vi "HFRR ADV v037 new software.vi"() -> ()   [LabVIEW 2025] (continued)
              n2898 = local write "Numeric 16"(w3970) -> ()
              n2899 = String Length(string=w3972) -> (length=w3975:i32)
              n2900 = Greater?(x=w3975, y=1) -> (0:w3971:bool)
            }
            n2901 = local write "String 29"(w3952) -> ()
            n2902 = Search and Replace String(input string=w3952, search string=".duf", replace string=".dgf" ("replace string (\"\")")) -> (result string=→"String Indicator 4":string)  [unwired: 5 in, 3 out]
            n2903 = Match Pattern(string=w3967, regular expression=".dwm") -> (before substring=w3951:string)  [unwired: 1 in, 3 out]
            "String Indicator" <- w3951
            n2904 = Match Pattern(string=w3952, regular expression=".dwm" ("substring (\"\")")) -> (before substring=w3953:string)  [unwired: 1 in, 3 out]
            "String Indicator 3" <- w3953
            n2905 = local write "TITTLE 2"(w3951) -> ()
            n2906 = String To Path(string=w3953) -> (path=w3960:path)
            "path" <- w3960
            n2907 = call <vilib>:"Read Characters From File.vi"("file path (dialog if empty)"=w3960, "start of read offset (chars.:0)"=60 ("start of read offset (chars.: 0)")) -> ("character string"=→"String Indicator 2":string)  [unwired: 4 in, 3 out]
          }
        }
        n2908 = call <vilib>:"Query Available Printers.vi"() -> ("system configured printers"=w3652:string[])  [unwired: 9 in, 2 out]
        "System Configured Printers 2" <- w3652
        n2909 = local read "OK Button 16"() -> (w3649:bool)
        n2910 = case shown="True" "OK Button 16" {
          frame False {
          }
          frame True {
            n2911 = stacked-sequence {
              frame #0 {
                n2912 = local read "Numeric 16"() -> (w3977:i32)
                n2913 = local write "Numeric 10"(w3977) -> ()
              }
              frame #1 {
                n2914 = local read "String 29"() -> (w3980:string)
                n2915 = String To Path(string=w3980) -> (path=w3979:path)
                n2916 = Open/Create/Replace File "Open File"(file path (use dialog)=w3979) -> (refnum out=w3981:refnum<file>)  [unwired: 5 in, 2 out]
                n2917 = for {
                  N: 16 -> [_]
                  tunnel: w3981 -> [w3988]
                  i -> [w3984]
                  (unwired) TRUE ("line mode (F)")
                  n2918 = Read from Text File "Read File"(file (use dialog)=w3988) -> (text=w3982:string)  [unwired: 3 in, 3 out]
                  n2919 = Match Pattern(string=w3982, regular expression="(") -> (after substring=w3987:string)  [unwired: 1 in, 3 out]
                  n2920 = Match Pattern(string=w3987, regular expression=")") -> (before substring=w3983:string)  [unwired: 1 in, 3 out]
                  n2921 = case shown="1" w3984 {
                    tunnel: w3983 -> [w3989 w3990 _ _ w3991 w3992 w3993 w3995 w3997 w3999 w4001 w4003 w4005 w4007 _]
                    tunnel: w3982 -> [_ _ _ _ _ _ _ _ _ _ _ _ _ _ _]
                    frame 0 {
                      "TITTLE" <- w3989
                    }
                    frame 1 {
                      "Sample ID" <- w3990
                    }
                    frame 2 {
                    }
                    frame 3 {
                    }
                    frame 4 {
                      "Test Date" <- w3991
                    }
                    frame 5 {
                      "Tested by" <- w3992
                    }
                    frame 6 {
                      n2922 = Fract/Exp String To Number(string=w3993) -> (number=→"Humidity before test 2":dbl)  [unwired: 3 in, 1 out]
                    }
                    frame 7 {
                      n2923 = Fract/Exp String To Number(string=w3995) -> (number=→"Temperature before test 2":dbl)  [unwired: 3 in, 1 out]
                    }
                    frame 8 {
                      n2924 = Fract/Exp String To Number(string=w3997) -> (number=→"Humidity after test 2":dbl)  [unwired: 3 in, 1 out]
                    }
                    frame 9 {
                      n2925 = Fract/Exp String To Number(string=w3999) -> (number=→"Temperature after test 2":dbl)  [unwired: 3 in, 1 out]
                    }
                    frame 10 {
                      n2926 = Fract/Exp String To Number(string=w4001) -> (number=→"MWSD 2":dbl)  [unwired: 3 in, 1 out]
                    }
                    frame 11 {
                      n2927 = Fract/Exp String To Number(string=w4003) -> (number=→"AVP 2":dbl)  [unwired: 3 in, 1 out]
                    }
                    frame 12 {
                      n2928 = Fract/Exp String To Number(string=w4005) -> (number=→"HCF 2":dbl)  [unwired: 3 in, 1 out]
                    }
                    frame 13 {
                      n2929 = Fract/Exp String To Number(string=w4007) -> (number=→"WS1.4 2":dbl)  [unwired: 3 in, 1 out]
                    }
                    frame 14, Default {
                    }
                  }
                }
              }
              frame #2 {
              }
            }
            n2930 = local write "OK Button 16"(FALSE ("OK Button 13")) -> ()
          }
        }
        n2931 = Index Array(array=w3652, index="Select Printer 3") -> (element=w3654:string)
        "Selected Printer" <- w3654
        n2932 = case shown="True" w3649 {
          frame False {
          }
          frame True {
            n2933 = flat-sequence {
              frame #0 {
              }
              frame #1 {
                n2934 = Wait (ms)(milliseconds to wait=u32 100) -> ()  [unwired: 1 out]
              }
              frame #2 {
                n2935 = local write "OK Button 16"(FALSE ("Print 3")) -> ()
              }
            }
          }
        }
        n2936 = case shown="True" "Print" {
          tunnel: w3654 -> [_ w3946]
          frame False {
          }
          frame True {
            (unwired) i16 6 ("width (-)")
            (unwired) "TESTED BY : "
            (unwired) "TESTED DATE :"
            (unwired) "SAMPLE ID : "
            (unwired) "SAMPLE DESIGN : "
            w3904 = "\r"
            w3921 = "\r"
            # "add image"
            n2937 = local read "Sample ID"() -> (w3894:string)
            n2938 = local read "Tested by"() -> (w3897:string)
            n2939 = local read "String 34"() -> (w3884:string)
            n2940 = local read "String 45"() -> (w3864:string)
            n2941 = local read "String 35"() -> (w3879:string)
            n2942 = local read "String 37"() -> (w3877:string)
            n2943 = local read "String 32"() -> (w3899:string)
            n2944 = local read "String 36"() -> (w3874:string)
            n2945 = local read "String 31"() -> (w3898:string)
            n2946 = local read "Test Date"() -> (w3895:string)
            n2947 = local read "String 33"() -> (w3900:string)
            n2948 = local read "String 38"() -> (w3870:string)
            n2949 = local read "String 39"() -> (w3867:string)
            n2950 = local write "Print"(FALSE ("Print FF")) -> ()
            n2951 = local read "S 39"() -> (w3882:string)
            n2952 = local read "S 38"() -> (w3889:string)
            n2953 = local read "Temperature before test 2"() -> (w3920:dbl)
            n2954 = local read "Temperature after test 2"() -> (w3910:dbl)
            n2955 = local read "Humidity before test 2"() -> (w3935:dbl)
            n2956 = local read "Humidity after test 2"() -> (w3919:dbl)
            n2957 = local read "MWSD 2"() -> (w3924:dbl)
            n2958 = local read "WS1.4 2"() -> (w3902:dbl)
            n2959 = Concatenate Strings("2)" ("string"), w3884) -> (w3885:string)
            n2960 = Concatenate Strings("3)" ("string"), w3882) -> (w3883:string)
            n2961 = Concatenate Strings("1)" ("string"), w3889) -> (w3888:string)
            n2962 = Concatenate Strings("4)" ("string"), w3879) -> (w3880:string)
            n2963 = Concatenate Strings("5)" ("string"), w3877) -> (w3876:string)
            n2964 = Concatenate Strings("6)" ("string"), w3874) -> (w3873:string)
            n2965 = Concatenate Strings("7)" ("string"), w3870) -> (w3871:string)
            n2966 = Concatenate Strings("8)" ("string"), w3867) -> (w3868:string)
            n2967 = local read "HCF 2"() -> (w3906:dbl)
            n2968 = local read "AVP 2"() -> (w3923:dbl)
            n2969 = local read "s.NO"() -> (w3865:string)
            n2970 = call <vilib>:"New Report.vi"("report type"=enum16{"Standard Report", "HTML"}."Standard Report") -> ("report out"=w3944:refnum<class "NI_report.lvclass">, "error out"=w3943:errorcluster)  [unwired: 13 in]
            n2971 = local read "TITTLE"() -> (w3896:string)
            n2972 = Concatenate Strings(w3921, w3864, w3865, w3921, w3899, w3894, w3921, w3898, w3895, w3921, w3900, w3897, w3921) -> (w3914:string)
            "test by" <- w3914
            n2973 = Number To Fractional String(number=w3920, width (-)=i16 6, precision (6)=i16 2) -> (F-format string=w3909:string)  [unwired: 1 in]
            n2974 = Number To Fractional String(number=w3919, width (-)=i16 6, precision (6)=i16 2) -> (F-format string=w3922:string)  [unwired: 1 in]
            n2975 = Number To Fractional String(number=w3935, width (-)=i16 6, precision (6)=i16 2) -> (F-format string=w3940:string)  [unwired: 1 in]
            n2976 = Number To Fractional String(number=w3924, width (-)=i16 6, precision (6)=i16 2) -> (F-format string=w3926:string)  [unwired: 1 in]
            n2977 = Number To Fractional String(number=w3910, width (-)=i16 6, precision (6)=i16 2) -> (F-format string=w3911:string)  [unwired: 1 in]
            n2978 = Number To Fractional String(number=w3923, width (-)=i16 6, precision (6)=i16 2) -> (F-format string=w3925:string)  [unwired: 1 in]
            n2979 = Number To Fractional String(number=w3906, width (-)=i16 6, precision (6)=i16 2) -> (F-format string=w3905:string)  [unwired: 1 in]
            n2980 = Number To Fractional String(number=w3902, precision (6)=i16 2) -> (F-format string=w3901:string)  [unwired: 2 in]
            n2981 = call-dynamic "Set Report Header Text.vi"("report in"=w3944, "center header text"=w3896, "error in (no error)"=w3943) -> ("report out"=w3915:refnum<class "NI_report.lvclass">, "error out"=w3916:errorcluster)  [unwired: 11 in]
            n2982 = Concatenate Strings(w3904, w3888, w3940, w3904, w3885, w3909, w3904, w3883, w3922, w3904, w3880, w3911, w3904, w3876, w3926, w3904, w3873, w3925, w3904, w3871, w3905, w3904, w3868, w3901) -> (w3892:string)
            "export 2" <- w3892
            n2983 = call-poly <vilib>:"Append Report Text.vi"("report in"=w3915, "text"=w3914, "error in (no error)"=w3916) -> ("report out"=w3918:refnum<class "NI_report.lvclass">, "error out"=w3917:errorcluster)  [unwired: 9 in, 2 out]
            n2984 = local read "test by"() -> (w3891:string)
            n2985 = local read "TITTLE"() -> (w3893:string)
            n2986 = call-poly <vilib>:"Append Report Text.vi"("report in"=w3918, "error in (no error)"=w3917) -> ("report out"=w3939:refnum<class "NI_report.lvclass">, "error out"=w3937:errorcluster)  [unwired: 10 in, 2 out]
            n2987 = Concatenate Strings(w3893, w3892, w3891) -> (→"output":string)
            n2988 = call-poly <vilib>:"Append Report Text.vi"("report in"=w3939, "text"=w3892, "error in (no error)"=w3937) -> ("report out"=w3938:refnum<class "NI_report.lvclass">, "error out"=w3936:errorcluster)  [unwired: 9 in, 2 out]
            n2989 = call-dynamic "Print Report.vi"("report in"=w3938, "printer name (default)"=w3946, "error in (no error)"=w3936) -> ("report out"=w3948:refnum<class "NI_report.lvclass">, "error out"=w3949:errorcluster)  [unwired: 11 in]
            n2990 = call-dynamic "Dispose Report.vi"("report in"=w3948, "error in (no error)"=w3949) -> ()  [unwired: 13 in, 1 out]
          }
        }
        n2991 = case shown="True" "Print 2" {
          frame False {
          }
          frame True {
            n2992 = flat-sequence {
              frame #0 {
                n2993 = local read "s.NO"() -> (→"s.NO 2":string)
                n2994 = Wait (ms)(milliseconds to wait=u32 20) -> ()  [unwired: 1 out]
                n2995 = local read "Sample ID  3"() -> (→"Sample ID  6":string)
                n2996 = local read "Sample ID  4"() -> (→"Sample ID  7":string)
                n2997 = local read "Sample ID"() -> (→"Sample ID  2":string)
                n2998 = local read "Tested by"() -> (→"Tested by 2":string)
                n2999 = local read "Test Date"() -> (→"Test Date 2":string)
                n3000 = local read "Humidity after test 3"() -> (→"Humidity after test 4":dbl)
                n3001 = local read "Ref A Test Date :"() -> (→"TITTLE 4":string)
                n3002 = local read "Temperature before test 3"() -> (w3771:dbl)
                n3003 = local read "Temperature before test 3"() -> (→"Temperature after test 5":dbl)
                n3004 = local read "Temperature after test 3"() -> (→"Temperature after test 4":dbl)
                n3005 = local read "Humidity before test 3"() -> (→"Humidity before test 4":dbl)
                n3006 = local write "Temperature before test 3"(w3771) -> ()
                n3007 = local read "image data"() -> (w3762:T16)
                n3008 = String To Path(string="C:\\LAB-IQ\\im\\Temp_resized.jpg") -> (path=w3763:path)
                "path 2" <- w3763
                n3009 = call <vilib>:"Write JPEG File.vi"("image data"=w3762, "path to JPEG file"=w3763) -> ()  [unwired: 8 in, 2 out]
                "Ref A Test Date :" <- "Ref A Test Date :"
                "Ref B Test Date :" <- "Ref B Test Date :"
                "Ref B Scar Value :" <- "Ref B Scar Value :"
                "Ref A Scar Value :" <- "Ref A Scar Value :"
              }
              frame #1 {
                (unwired) HTML_Report_Image_Alignment."MIDDLE" ("alignment (default)")
                w3799 = u16 0 items=["portrait", "landscape"] ("orientation (portrait)")
                (unwired) HTML_Report_Image_Alignment."ABSMIDDLE" ("alignment (default)")
                (unwired) "TESTED BY : "
                (unwired) "TESTED DATE :"
                (unwired) "SAMPLE ID : "
                (unwired) "SAMPLE DESIGN : "
                w3832 = "\r"
                # "add image"
                n3010 = Wait (ms)(milliseconds to wait=u32 20) -> ()  [unwired: 1 out]
                n3011 = local read "Sample ID  2"() -> (w3825:string)
                n3012 = local read "Wear Scar X"() -> (w3797:dbl)
                "Length ( microns ) 2" <- w3797
                n3013 = local read "Wear Scar Y"() -> (w3796:dbl)
                "Wear Scar Y ( microns ) :" <- w3796
                n3014 = local read "Test Date 2"() -> (w3826:string)
                n3015 = local read "Tested by 2"() -> (w3827:string)
                n3016 = local read "String 46"() -> (w3823:string)
                n3017 = local read "String 48"() -> (w3829:string)
                n3018 = local read "String 47"() -> (w3828:string)
                n3019 = local read "String 49"() -> (w3830:string)
                n3020 = local read "String 10"() -> (w3783:string)
                n3021 = local read "s.NO 2"() -> (w3824:string)
                n3022 = Add(x=w3797, y=w3796) -> (x+y=w3795:dbl)
                n3023 = call <vilib>:"New Report.vi"("report type"=enum16{"Standard Report", "HTML"}."HTML") -> ("report out"=w3803:refnum<class "NI_report.lvclass">, "error out"=w3801:errorcluster)  [unwired: 13 in]
                n3024 = Concatenate Strings(w3832, w3823, w3824, w3832, w3829, w3825, w3832, w3828, w3826, w3832, w3830, w3827, w3832) -> (→"test by 2":string)
                n3025 = Concatenate Strings("C:\\LAB-IQ\\Data\\" ("string"), w3783, ".jpg" ("string")) -> ()  [unwired: 1 out]
                n3026 = Divide(x=w3795, y=2.0) -> (x/y=→"Mean Wear ( microns) :":dbl)
                n3027 = call-dynamic "Set Report Orientation.vi"("report in"=w3803, "orientation (portrait)"=w3799, "error in (no error)"=w3801) -> ("report out"=w3802:refnum<class "NI_report.lvclass">, "error out"=w3800:errorcluster)  [unwired: 11 in]
                n3028 = for {
                  N: 5 -> [_]
                  tunnel: w3802 -> [w3853]
                  tunnel: [w3852] -> w3781
                  tunnel: w3800 -> [w3851]
                  tunnel: [w3850] -> w3780
                  n3029 = call-dynamic "Set Report Tab Width.vi"("report in"=w3853, "error in (no error)"=w3851) -> ("report out"=w3852:refnum<class "NI_report.lvclass">, "error out"=w3850:errorcluster)  [unwired: 12 in]
                }
                n3030 = local read "TITTLE"() -> (w3798:string)
                n3031 = call-dynamic "Set Report Header Text.vi"("report in"=w3781, "center header text"=w3798, "error in (no error)"=w3780) -> ("report out"=w3819:refnum<class "NI_report.lvclass">, "error out"=w3818:errorcluster)  [unwired: 11 in]
                n3032 = for {
                  N: 1 -> [_]
                  tunnel: [w3857] -> w3805
                  tunnel: [w3856] -> w3804
                  tunnel: w3819 -> [w3855]
                  tunnel: w3818 -> [w3854]
                  n3033 = call-dynamic "New Report Line.vi"("report in"=w3855, "error in (no error)"=w3854) -> ("report out"=w3857:refnum<class "NI_report.lvclass">, "error out"=w3856:errorcluster)  [unwired: 12 in]
                }
                n3034 = for {
                  N: 2 -> [_]
                  tunnel: [w3849] -> w3811
                  tunnel: [w3848] -> w3810
                  tunnel: w3805 -> [w3847]
                  tunnel: w3804 -> [w3846]
                  n3035 = call-dynamic "New Report Line.vi"("report in"=w3847, "error in (no error)"=w3846) -> ("report out"=w3849:refnum<class "NI_report.lvclass">, "error out"=w3848:errorcluster)  [unwired: 12 in]
                }
                n3036 = for {
                  N: 25 -> [_]
                  tunnel: w3811 -> [w3845]
                  tunnel: w3810 -> [w3843]
                  tunnel: [w3844] -> w3814
                  tunnel: [w3842] -> w3813
                  n3037 = call-dynamic "Set Report Tab Width.vi"("report in"=w3845, "error in (no error)"=w3843) -> ("report out"=w3844:refnum<class "NI_report.lvclass">, "error out"=w3842:errorcluster)  [unwired: 12 in]
                }
                n3038 = control-ref of="Tab Control 9"() -> (w3809:refnum<vi>)
                n3039 = call-dynamic "Append Control Image to Report.vi"("report in"=w3814, "alignment (default)"=HTML_Report_Image_Alignment."ABSMIDDLE", "ctrl reference"=w3809, "error in (no error)"=w3813) -> ("report out"=w3808:refnum<class "NI_report.lvclass">, "error out"=w3807:errorcluster)  [unwired: 8 in, 2 out]
                n3040 = for {
                  N: 3 -> [_]
                  tunnel: [w3841] -> w3792
                  tunnel: [w3840] -> w3791
                  tunnel: w3808 -> [w3839]
                  tunnel: w3807 -> [w3838]
                  n3041 = call-dynamic "New Report Line.vi"("report in"=w3839, "error in (no error)"=w3838) -> ("report out"=w3841:refnum<class "NI_report.lvclass">, "error out"=w3840:errorcluster)  [unwired: 12 in]
                }
                n3042 = for {
                  N: 100 -> [_]
                  tunnel: w3792 -> [w3837]
                  tunnel: w3791 -> [w3835]
                  tunnel: [w3836] -> w3788
                  tunnel: [w3834] -> w3786
                  n3043 = call-dynamic "Set Report Tab Width.vi"("report in"=w3837, "error in (no error)"=w3835) -> ("report out"=w3836:refnum<class "NI_report.lvclass">, "error out"=w3834:errorcluster)  [unwired: 12 in]
                }
                n3044 = String To Path(string="C:\\LAB-IQ\\im\\Temp_resized.jpg") -> (path=w3778:path)
                n3045 = call-poly <vilib>:"Append Image to Report.vi"("report in"=w3788, "path or URL of image"=w3778, "error in (no error)"=w3786) -> ("report out"=w3787:refnum<class "NI_report.lvclass">, "error out"=w3785:errorcluster)  [unwired: 9 in, 2 out]
                n3046 = call-poly <vilib>:"Open HTML Report in Browser.vi"("report in"=w3787, "error in (no error)"=w3785) -> ("report out"=w3822:refnum<class "NI_report.lvclass">, "error out"=w3821:errorcluster)  [unwired: 11 in, 1 out]
                n3047 = call-dynamic "Dispose Report.vi"("report in"=w3822, "error in (no error)"=w3821) -> ()  [unwired: 13 in, 1 out]
              }
              frame #2 {
              }
              frame #3 {
                n3048 = disable-structure shown="Disabled" {
                  frame Disabled {
                    n3049 = local read "String 10"() -> (w3862:string)
                    n3050 = Concatenate Strings("C:\\LAB-IQ-NXT\\Data\\" ("string"), w3862, ".jpg" ("string")) -> (w3860:string)
                    n3051 = String To Path(string=w3860) -> (path=w3859:path)
                    n3052 = Delete(path (use dialog)=w3859) -> ()  [unwired: 4 in, 3 out]
                  }
                  frame Enabled {
                  }
                }
                n3053 = local write "Print 2"(FALSE ("Print")) -> ()
              }
            }
          }
        }
      }
    }
    n3054 = Wait (ms)(milliseconds to wait=u32 50) -> ()  [unwired: 1 out]
    n3055 = Wait (ms)(milliseconds to wait=u32 50) -> ()  [unwired: 1 out]
    n3056 = local read "Quit"() -> (w2196:bool)
  }
  n3057 = VISA Close(VISA resource name=w41, error in (no error)=w40) -> ()  [unwired: 1 out]
  n3058 = while {
    stop <- w4013 stop-if-true
    n3059 = local read "Auto Start Test"() -> (w4011:bool)
    n3060 = local read "RUN"() -> (w4010:bool)
    n3061 = Wait (ms)(milliseconds to wait=u32 1000) -> ()  [unwired: 1 out]
    n3062 = Or(x=w4010, y=w4011) -> (x .or. y?=w4009:bool)
    n3063 = case shown="True" w4009 {
      frame False {
      }
      frame True {
        n3064 = local read "LVDT STROKE Actual"() -> (w4014:dbl)
        n3065 = In Range and Coerce(upper limit=1.2, x=w4014, lower limit=0.6) -> (In Range?=w4017:bool)  [unwired: 1 out]
        n3066 = call-poly <vilib>:"Random Number (Range).vi"("lower bound (0)"=0.998 ("upper bound (100)"), "upper bound (100)"=1.003) -> ("number"=w4015:dbl)  [unwired: 9 in]
        n3067 = case shown="True" w4017 {
          tunnel: [w4022 w4023] -> w4016
          tunnel: w4015 -> [_ w4023]
          tunnel: w4014 -> [w4022 _]
          frame False {
          }
          frame True {
          }
        }
        "LVDT STROKE DISPLAY" <- w4016
      }
    }
    n3068 = local read "Quit"() -> (w4013:bool)
  }
  n3069 = while {
    tunnel: [w4040] -> w49
    shift-right: [w4033] -> _
    shift-left: 0.0 -> [w4036]
    shift-right: [w4032] -> _
    shift-left: 0.0 -> [w4035]
    shift-right: [w4031] -> _
    shift-left: 100.0 ("vc_cmd") -> [w4034]
    stop <- w4040 stop-if-true
    # "PID LOGIC"
    n3070 = local read "run test Calibration"() -> (w4028:bool)
    n3071 = local read "RUN"() -> (w4038:bool)
    n3072 = local read "Auto Start Temp"() -> (w4029:bool)
    n3073 = local read "Auto Start Test"() -> (w4037:bool)
    n3074 = local read "START TEMP"() -> (w4027:bool)
    n3075 = And(x=w4029, y=w4037) -> (x .and. y?=w4030:bool)
    n3076 = Or(x=w4038, y=w4030) -> (x .or. y?=w4039:bool)
    n3077 = And(x=w4039, y=w4027) -> (x .and. y?=w4026:bool)
    n3078 = And(x=w4028, y=w4027) -> (x .and. y?=w4025:bool)
    n3079 = Or(x=w4025, y=w4026) -> (x .or. y?=w4024:bool)
    n3080 = Wait (ms)(milliseconds to wait="milliseconds to wait") -> ()  [unwired: 1 out]
    n3081 = case shown="True" w4024 {
      tunnel: [400.0 ("out_vc_cmd") w4059] -> w4031
      tunnel: [w4043 w4061] -> w4032
      tunnel: [w4043 w4060] -> w4033
      tunnel: w4036 -> [_ w4050]
      tunnel: w4035 -> [_ w4049]
      tunnel: w4034 -> [_ w4048]
      tunnel: w4028 -> [_ w4044]
      frame False {
        w4043 = 0.0 ("error_out")
      }
      frame True {
        n3082 = case shown="True" w4044 {
          tunnel: [w4068 1.0] -> w4046
          frame False {
            n3083 = local read "Set Strk"() -> (w4067:dbl)
            n3084 = Add(x=w4067, y="Add up Stroke") -> (x+y=w4068:dbl)
          }
          frame True {
          }
        }
        n3085 = local read "LVDT STROKE"() -> (w4045:dbl)
        n3086 = formula code="// Zero-Hardcode Explicit Positional-Form PID Engine\n// Inputs: target_stroke, measured_stroke, dt, prev_error, integral_accumulator_in, prev_vc_cmd\n//         kp, ki, kd, max_step_change, max_amplitude, min_amplitude, startup_cmd\n// Outputs: vc_cmd, error_out, out_error, integral_accumulator_out, out_vc_cmd\n\n// 1. Calculate Tracking Error\nfloat current_error = target_stroke - measured_stroke;\nerror_out = current_error;\n\n// 2. Compute Proportional Term\nfloat p_term = kp * current_error;\n\n// 3. Compute Derivative Term\nfloat d_term = 0.0;\nif (dt > 0.0) {\n    d_term = kd * ((current_error - prev_error) / dt);\n}\n\n// 4. Update and Accumulate Integral Term\nfloat current_integral = integral_accumulator_in + (current_error * dt);\nfloat i_term = ki * current_integral;\n\n// 5. Calculate Ideal Target Command (Anchored by startup baseline)\nfloat ideal_command = startup_cmd + p_term + i_term + d_term;\n\n// 6. Apply Loop Rate Limiting FIRST \n// (Forces the command to climb gradually from prev_vc_cmd instead of jumping straight to max)\nfloat raw_adjustment = ideal_command - prev_vc_cmd;\n\nif (raw_adjustment > max_step_change) {\n    raw_adjustment = max_step_change;\n} else if (raw_adjustment < -max_step_change) {\n    raw_adjustment = -max_step_change;\n}\n\nfloat next_vc_cmd = prev_vc_cmd + raw_adjustment;\n\n// 7. Anti-Windup Protection & Final Output Safety Safeguard Clamping\n// (Back-calculating based on what we are ACTUALLY outputting)\nif (next_vc_cmd > max_amplitude) {\n    float excess = next_vc_cmd - max_amplitude;\n    if (ki > 0.0) {\n        current_integral -= excess / ki;\n    }\n    next_vc_cmd = max_amplitude;\n} else if (next_vc_cmd < min_amplitude) {\n    float excess = next_vc_cmd - min_amplitude;\n    if (ki > 0.0) {\n        current_integral -= excess / ki;\n    }\n    next_vc_cmd = min_amplitude;\n}\n\n// 8. Map to Shift Registers for memory persistence\nvc_cmd = next_vc_cmd;\nout_error = current_error;                   \nintegral_accumulator_out = current_integral;  \nout_vc_cmd = next_vc_cmd;"("target_stroke"=w4046, "measured_stroke"=w4045, "dt"="dt", "integral_accumulator_in"=w4049, "prev_error"=w4050, "prev_vc_cmd"=w4048, "kp"="kp", "ki"="ki", "kd"="kd", "max_step_change"="max_step_change", "max_amplitude"="max_amplitude", "min_amplitude"="min_amplitude", "startup_cmd"="startup_cmd") -> ("vc_cmd"=w4065:dbl, "out_error"=w4060:dbl, "integral_accumulator_out"=w4061:dbl, "out_vc_cmd"=w4059:dbl)  [unwired: 1 out]
        "output Vpp" <- w4065
        n3087 = Number To Fractional String(number=w4065, precision (6)=i16 1) -> (F-format string=w4063:string)  [unwired: 2 in]
        n3088 = Concatenate Strings("DAC;" ("string"), w4063) -> (w4047:string)
        n3089 = local write "Due Write"(w4047) -> ()
        "prev_error" <- w4050
        "integral_accumulator_in" <- w4049
        "prev_vc_cmd" <- w4048
      }
    }
    n3090 = local read "Quit"() -> (w4040:bool)
  }
  n3091 = Or(x=w45, y=w44) -> (x .or. y?=w46:bool)
  n3092 = Or(x=w42, y=w46) -> (x .or. y?=w51:bool)
  n3093 = control-ref of="new picture"() -> ()  [unwired: 1 out]
  n3094 = Or(x=w54, y=w51) -> (x .or. y?=w48:bool)
  n3095 = Or(x=w48, y=w49) -> (x .or. y?=w43:bool)
  n3096 = while {
    tunnel: [w4070] -> w53
    i -> [w4077]
    stop <- w4070 stop-if-true
    n3097 = local read "Quit"() -> (w4070:bool)
    n3098 = Equal To 0?(x=w4077) -> (x = 0?=w4075:bool)
    n3099 = call "Elapsed Time3"("Time Target (s)"=45.0, "Auto Reset"=TRUE) -> ("Time has Elapsed"=w4074:bool)  [unwired: 10 in, 7 out]
    n3100 = Wait (ms)(milliseconds to wait=u32 50) -> ()  [unwired: 1 out]
    n3101 = Or(x=w4074, y=w4075) -> (x .or. y?=w4076:bool)
    n3102 = case shown="True" w4076 {
      frame False {
      }
      frame True {
        n3103 = call <vilib>:"System Exec.vi"("run minimized? (F)"=TRUE, "error in (no error)"="error in (no error)", "command line"="powercfg.exe -change -monitor-timeout-ac 0") -> ("error out"=w4088:errorcluster)  [unwired: 5 in, 3 out]
        n3104 = call <vilib>:"System Exec.vi"("run minimized? (F)"=TRUE, "error in (no error)"=w4088, "command line"="powercfg.exe -change -disk-timeout-ac 0") -> ("error out"=w4087:errorcluster)  [unwired: 5 in, 3 out]
        n3105 = call <vilib>:"System Exec.vi"("run minimized? (F)"=TRUE, "error in (no error)"=w4087, "command line"="powercfg.exe -change -standby-timeout-ac 0") -> ("error out"=w4086:errorcluster)  [unwired: 5 in, 3 out]
        n3106 = call <vilib>:"System Exec.vi"("run minimized? (F)"=TRUE, "error in (no error)"=w4086, "command line"="powercfg.exe -change -hibernate-timeout-ac 0") -> ("error out"=w4085:errorcluster)  [unwired: 5 in, 3 out]
        n3107 = call <vilib>:"Simple Error Handler.vi"("error in (no error)"=w4085) -> ("error out"=w4091:errorcluster)  [unwired: 4 in, 4 out]
        n3108 = call <vilib>:"Clear Errors.vi"("error in (no error)"=w4091) -> ("error out"=→"error out":errorcluster)  [unwired: 5 in, 1 out]
      }
    }
  }
  n3109 = Compound Arithmetic op=OR(w56, w43, w53) -> (w55:bool)
  n3110 = flat-sequence {
    tunnel: w55 -> [_]
    tunnel: [w4093] -> w25
    tunnel: w25 -> [_]
    frame #0 {
      n3111 = call "CLOSE CONNECTION.vi"() -> ("error out"=w4093:errorcluster)  [unwired: 11 in]
    }
    frame #1 {
      n3112 = Quit LabVIEW(quit? (T)=TRUE) -> ()
      n3113 = local write "Quit"(FALSE ("EXIT")) -> ()
    }
  }
  n3114 = property on="Heater Button" class="Bool (strict)"("Visible"=TRUE) -> ()  [unwired: 2 in, 2 out]
  n3115 = while {
    tunnel: [w4100] -> _
    i -> [w4100]
    stop <- w4096 stop-if-true
    # "Langauage selection"
    n3116 = Equal?(x="Lan flag", y=22.0) -> ()  [unwired: 1 out]
    n3117 = disable-structure shown="Disabled" {
      frame Disabled {
        n3118 = stacked-sequence {
          frame #0 {
            n3119 = case shown="\"Russian\"" "Language Selection" {
              tunnel: [0 1] -> w4102
              frame "English", Default {
              }
              frame "Russian" {
              }
            }
            n3120 = for {
              N: 130 -> [_]
              tunnel: "Table" -> [w4111]
              tunnel: w4102 -> [w4110]
              i -> [w4109]
              n3121 = Index Array(array=w4111, index (row)=w4109, index (col)=w4110) -> (element=w4108:string)
              n3122 = case shown="1" w4109 {
                tunnel: w4108 -> [w4112 w4113 _ w4114 w4115 w4116 w4117 w4118 w4119 w4120 w4121 w4122 w4123 w4124 w4125 w4126 w4127 w4128 w4129 w4130 w4131 w4132 w4133 w4134 w4135 w4136 w4137 w4138 w4139 _ _ w4140 w4141 w4142 w4143 w4144 w4145 w4154 w4161 w4168 w4175 w4179 w4182 w4185 w4187 w4189 w4190 w4191 w4192 w4193 w4194 w4195 w4196 w4197 w4198 w4199 w4200 w4201 w4202 w4203 w4204 w4205 w4206 w4207 w4208 w4209 w4210 w4211 w4212 w4213 w4214 w4215 w4216 w4217 w4218 w4219 w4220 w4221 w4222 w4223 w4224 w4225 w4226 w4227 w4228 w4229 w4230 w4231 w4232 w4233 w4234 w4235 w4236 w4237 w4238 w4239 w4240 w4241 w4242 w4243 w4244 w4245 w4246 w4247 w4248 _ w4249 w4250 w4251 w4252 w4253 w4254 w4255 w4256 w4257 w4258 w4259 w4260 w4261 _ w4262 w4263 w4264 w4265 w4266 w4267 _]
                frame 0 {
                  n3123 = local write "S"(w4112) -> ()
                }
                frame 1 {
                  n3124 = local write "S 2"(w4113) -> ()
                }
                frame 2 {
                }
                frame 3 {
                  n3125 = local write "S 4"(w4114) -> ()
                }
                frame 4 {
                  n3126 = property on="FILE" class="Str"("Caption.Text"=w4115) -> ()  [unwired: 2 in, 2 out]
                }
                frame 5 {
                  n3127 = property on="Fuel Discription :" class="Str"("Caption.Text"=w4116) -> ()  [unwired: 2 in, 2 out]
                }
                frame 6 {
                  n3128 = property on="Remarks :" class="Str"("Caption.Text"=w4117) -> ()  [unwired: 2 in, 2 out]
                }
                frame 7 {
                  n3129 = property on="Save & Continue" class="Bool (strict)"("Boolean Text.Text"=w4118) -> ()  [unwired: 2 in, 2 out]
                }
                frame 8 {
                }
                frame 9 {
                  n3130 = property on="Set Hz" class="DigNum (strict)"("Caption.Text"=w4120) -> ()  [unwired: 2 in, 2 out]
                }
                frame 10 {
                }
                frame 11 {
                  n3131 = property on="NORMAL LOAD" class="DigNum (strict)"("Caption.Text"=w4122) -> ()  [unwired: 2 in, 2 out]
                }
                frame 12 {
                }
                frame 13 {
                  n3132 = property on="Set Temp" class="DigNum (strict)"("Caption.Text"=w4124) -> ()  [unwired: 2 in, 2 out]
                }
                frame 14 {
                  n3133 = local write "S 15"(w4125) -> ()
                }
                frame 15 {
                  n3134 = property on="Set Rh" class="DigNum (strict)"("Caption.Text"=w4126) -> ()  [unwired: 2 in, 2 out]
                }
                frame 16 {
                }
                frame 17 {
                  n3135 = local write "S 18"(w4128) -> ()
                }
                frame 18 {
                  "String 17" <- w4129
                }
                frame 19 {
                  n3136 = property on="test time" class="DigNum (strict)"("Caption.Text"=w4130) -> ()  [unwired: 2 in, 2 out]
                }
                frame 20 {
                  "String 18" <- w4131
                  "String 22" <- w4131
                }
                frame 21 {
                  n3137 = property on="Elapsed time" class="DigNum (strict)"("Caption.Text"=w4132) -> ()  [unwired: 2 in, 2 out]
                }
                frame 22 {
                  n3138 = property on="Samplingtime 2" class="DigNum (strict)"("Caption.Text"=w4133) -> ()  [unwired: 2 in, 2 out]
                }
                frame 23 {
                  "String 21" <- w4134
                }
                frame 24 {
                  n3139 = property on="Countdown" class="DigNum (strict)"("Caption.Text"=w4135) -> ()  [unwired: 2 in, 2 out]
                }
                frame 25 {
                  n3140 = property on="Countdown 2" class="DigNum (strict)"("Caption.Text"=w4136) -> ()  [unwired: 2 in, 2 out]
                }
                frame 26 {
                  n3141 = property on="Engage" class="Bool (strict)"("Boolean Text.Text"=w4137) -> ()  [unwired: 2 in, 2 out]
                }
                frame 27 {
                  n3142 = property on="Boolean  4" class="Bool (strict)"("Boolean Text.Text"=w4138) -> ()  [unwired: 2 in, 2 out]
                }
                frame 28 {
                  n3143 = property on="Test \nStatus" class="Bool (strict)"("Boolean Text.Text"=w4139) -> ()  [unwired: 2 in, 2 out]
                }
                frame 29 {
                }
                frame 30 {
                }
                frame 31 {
                }
                frame 32 {
                  n3144 = property on="RSTCOF" class="Bool"("Boolean Text.Text"=w4141) -> ()  [unwired: 2 in, 2 out]
                  n3145 = property on="RST FF" class="Bool"("Boolean Text.Text"=w4141) -> ()  [unwired: 2 in, 2 out]
                  n3146 = property on="RST TEMP" class="Bool"("Boolean Text.Text"=w4141) -> ()  [unwired: 2 in, 2 out]
                  n3147 = property on="RSTV1 3" class="Bool"("Boolean Text.Text"=w4141) -> ()  [unwired: 2 in, 2 out]
                  n3148 = property on="rstv2" class="Bool"("Boolean Text.Text"=w4141) -> ()  [unwired: 2 in, 2 out]
                  n3149 = property on="RSTV1 2" class="Bool"("Boolean Text.Text"=w4141) -> ()  [unwired: 2 in, 2 out]
                  n3150 = property on="RST CP" class="Bool"("Boolean Text.Text"=w4141) -> ()  [unwired: 2 in, 2 out]
                }
                frame 33 {
                  "S 61" <- w4142
                }
                frame 34 {
                  "String 23" <- w4143
                }
                frame 35 {
                  n3151 = property on="Rh Before" class="DigNum (strict)"("Caption.Text"=w4144) -> ()  [unwired: 2 in, 2 out]
                }
                frame 36 {
                  n3152 = Match Pattern(string=w4145, regular expression=",") -> (before substring=→"bs":string, after substring=→"as":string)  [unwired: 1 in, 2 out]
                  n3153 = property on="Rh After" class="DigNum (strict)"("Caption.Text"=w4145) -> ()  [unwired: 2 in, 2 out]
                }
                frame 37 {
                  n3154 = Match Pattern(string=w4154, regular expression=",") -> (before substring=w4153:string, after substring=w4152:string)  [unwired: 1 in, 2 out]
                  "bs" <- w4153
                  "as" <- w4152
                  n3155 = Concatenate Strings(w4153, w4152) -> (w4149:string)
                  n3156 = property on="Humidity before test 2" class="DigNum (strict)"("Caption.Text"=w4149) -> ()  [unwired: 2 in, 2 out]
                  n3157 = Concatenate Strings(w4149, "=" ("string")) -> (w4150:string)
                  n3158 = local write "S 38"(w4150) -> ()
                }
                frame 38 {
                  n3159 = Match Pattern(string=w4161, regular expression=",") -> (before substring=w4160:string, after substring=w4159:string)  [unwired: 1 in, 2 out]
                  "bs" <- w4160
                  "as" <- w4159
                  n3160 = Concatenate Strings(w4160, w4159) -> (w4156:string)
                  n3161 = property on="Humidity after test 2" class="DigNum (strict)"("Caption.Text"=w4156) -> ()  [unwired: 2 in, 2 out]
                  n3162 = Concatenate Strings(w4156, "=" ("string")) -> (w4158:string)
                  n3163 = local write "S 39"(w4158) -> ()
                }
                frame 39 {
                  n3164 = Match Pattern(string=w4168, regular expression=",") -> (before substring=w4167:string, after substring=w4166:string)  [unwired: 1 in, 2 out]
                  "bs" <- w4167
                  "as" <- w4166
                  n3165 = Concatenate Strings(w4167, w4166) -> (w4163:string)
                  n3166 = property on="Temperature before test 2" class="DigNum (strict)"("Caption.Text"=w4163) -> ()  [unwired: 2 in, 2 out]
                  n3167 = Concatenate Strings(w4163, "=" ("string")) -> (→"String 34":string)
                }
                frame 40 {
                  n3168 = Match Pattern(string=w4175, regular expression=",") -> (before substring=w4174:string, after substring=w4173:string)  [unwired: 1 in, 2 out]
                  "bs" <- w4174
                  "as" <- w4173
                  n3169 = Concatenate Strings(w4174, w4173) -> (w4170:string)
                  n3170 = property on="Temperature after test 2" class="DigNum (strict)"("Caption.Text"=w4170) -> ()  [unwired: 2 in, 2 out]
                  n3171 = Concatenate Strings(w4170, "=" ("string")) -> (→"String 35":string)
                  n3172 = property on="Temperature after test" class="DigNum (strict)"("Caption.Text"=w4170) -> ()  [unwired: 2 in, 2 out]
                }
                frame 41 {
                  n3173 = property on="AVP 2" class="DigNum (strict)"("Caption.Text"=w4179) -> ()  [unwired: 2 in, 2 out]
                  n3174 = Concatenate Strings(w4179, "=" ("string")) -> (→"String 36":string)
                }
                frame 42 {
                  n3175 = property on="MWSD 2" class="DigNum (strict)"("Caption.Text"=w4182) -> ()  [unwired: 2 in, 2 out]
                  n3176 = Concatenate Strings(w4182, "=" ("string")) -> (→"String 37":string)
                }
                frame 43 {
                  n3177 = property on="HCF 2" class="DigNum (strict)"("Caption.Text"=w4185) -> ()  [unwired: 2 in, 2 out]
                  n3178 = Concatenate Strings(w4185, "=" ("string")) -> (→"String 38":string)
                }
                frame 44 {
                  n3179 = Concatenate Strings(w4187, "=" ("string")) -> (→"String 39":string)
                  n3180 = property on="WS1.4 2" class="DigNum (strict)"("Caption.Text"=w4187) -> ()  [unwired: 2 in, 2 out]
                }
                frame 45 {
                }
                frame 46 {
                  n3181 = local write "S 47"(w4190) -> ()
                }
                frame 47 {
                  n3182 = local write "S 48"(w4191) -> ()
                }
                frame 48 {
                  n3183 = local write "S 49"(w4192) -> ()
                }
                frame 49 {
                  n3184 = local write "S 50"(w4193) -> ()
                }
                frame 50 {
                  n3185 = local write "S 51"(w4194) -> ()
                }
                frame 51 {
                  n3186 = local write "S 52"(w4195) -> ()
                }
                frame 52 {
                  n3187 = local write "S 53"(w4196) -> ()
                }
                frame 53 {
                  n3188 = local write "S 54"(w4197) -> ()
                }
                frame 54 {
                  n3189 = local write "S 55"(w4198) -> ()
                }
                frame 55 {
                  n3190 = local write "S 56"(w4199) -> ()
                }
                frame 56 {
                  n3191 = local write "S 57"(w4200) -> ()
                }
                frame 57 {
                  n3192 = local write "S 58"(w4201) -> ()
                }
                frame 58 {
                  n3193 = local write "S 59"(w4202) -> ()
                }
                frame 59 {
                  n3194 = local write "S 60"(w4203) -> ()
                }
                frame 60 {
                  n3195 = local write "S 62"(w4204) -> ()
                }
                frame 61 {
                  n3196 = local write "S 63"(w4205) -> ()
                }
                frame 62 {
                  n3197 = local write "S 64"(w4206) -> ()
                }
                frame 63 {
                  n3198 = local write "S 65"(w4207) -> ()
                }
                frame 64 {
                  n3199 = local write "S 66"(w4208) -> ()
                }
                frame 65 {
                  n3200 = local write "S 67"(w4209) -> ()
                }
                frame 66 {
                  n3201 = local write "S 68"(w4210) -> ()
                }
                frame 67 {
                  n3202 = local write "S 69"(w4211) -> ()
                }
                frame 68 {
                  n3203 = local write "S 70"(w4212) -> ()
                }
                frame 69 {
                  n3204 = local write "S 71"(w4213) -> ()
                }
                frame 70 {
                  n3205 = local write "S 72"(w4214) -> ()
                }
                frame 71 {
                  n3206 = local write "S 73"(w4215) -> ()
                }
                frame 72 {
                  n3207 = local write "S 74"(w4216) -> ()
                }
                frame 73 {
                  n3208 = local write "S 75"(w4217) -> ()
                }
                frame 74 {
                  n3209 = local write "S 76"(w4218) -> ()
                }
                frame 75 {
                  n3210 = local write "S 77"(w4219) -> ()
                }
                frame 76 {
                  n3211 = local write "S 78"(w4220) -> ()
                }
                frame 77 {
                  n3212 = local write "S 79"(w4221) -> ()
                }
                frame 79 {
                  n3213 = property on="Sample Temperature ( °C )" class="XYGraph (strict)"("Y Scale.Name Label.Text"=w4222) -> ()  [unwired: 2 in, 2 out]
                }
                frame 80 {
                  n3214 = local write "S 81"(w4223) -> ()
                  n3215 = property on="Humidity ( %RH )" class="XYGraph (strict)"("Y Scale.Name Label.Text"=w4223) -> ()  [unwired: 2 in, 2 out]
                }
                frame 78 {
                  n3216 = property on="Air Temperature  ( °C )" class="XYGraph (strict)"("X Scale.Name Label.Text"=w4224) -> ()  [unwired: 2 in, 2 out]
                  n3217 = property on="Humidity ( %RH )" class="XYGraph (strict)"("X Scale.Name Label.Text"=w4224) -> ()  [unwired: 2 in, 2 out]
                  n3218 = property on="Sample Temperature ( °C )" class="XYGraph (strict)"("X Scale.Name Label.Text"=w4224) -> ()  [unwired: 2 in, 2 out]
                  n3219 = property on="Coefficient Of Friction" class="XYGraph (strict)"("X Scale.Name Label.Text"=w4224) -> ()  [unwired: 2 in, 2 out]
                }
                frame 81 {
                  n3220 = property on="Air Temperature  ( °C )" class="XYGraph (strict)"("Y Scale.Name Label.Text"=w4225) -> ()  [unwired: 2 in, 2 out]
                }
                frame 82 {
                  n3221 = local write "S 84"(w4226) -> ()
                }
                frame 83 {
                  n3222 = local write "S 85"(w4227) -> ()
                }
                frame 84 {
                  n3223 = local write "S 86"(w4228) -> ()
                }
                frame 85 {
                  n3224 = local write "S 87"(w4229) -> ()
                }
                frame 86 {
                  n3225 = local write "S 88"(w4230) -> ()
                }
                frame 87 {
                }
                frame 88 {
                  n3226 = local write "S 90"(w4232) -> ()
                }
                frame 89 {
                  n3227 = local write "S 91"(w4233) -> ()
                }
                frame 90 {
                  n3228 = local write "S 92"(w4234) -> ()
                }
                frame 91 {
                  n3229 = local write "S 93"(w4235) -> ()
                }
                frame 92 {
                  n3230 = local write "S 94"(w4236) -> ()
                }
                frame 93 {
                  n3231 = local write "S 95"(w4237) -> ()
                }
                frame 94 {
                  n3232 = local write "S 96"(w4238) -> ()
                }
                frame 95 {
                  n3233 = local write "S 97"(w4239) -> ()
                }
                frame 96 {
                  n3234 = local write "S 98"(w4240) -> ()
                }
                frame 97 {
                  n3235 = local write "S 99"(w4241) -> ()
                }
                frame 98 {
                  n3236 = local write "S 100"(w4242) -> ()
                }
                frame 99 {
                  n3237 = local write "S 101"(w4243) -> ()
                }
                frame 100 {
                  n3238 = local write "S 102"(w4244) -> ()
                }
                frame 101 {
                  n3239 = local write "S 103"(w4245) -> ()
                }
                frame 102 {
                  n3240 = local write "S 104"(w4246) -> ()
                }
                frame 103 {
                  n3241 = local write "S 105"(w4247) -> ()
                }
                frame 104 {
                  n3242 = local write "S 106"(w4248) -> ()
                }
                frame 105 {
                }
                frame 106 {
                  n3243 = property on="OK Button 17" class="Bool (strict)"("Boolean Text.Text"=w4249) -> ()  [unwired: 2 in, 2 out]
                }
                frame 107 {
                  n3244 = property on="OK Button 16" class="Bool (strict)"("Boolean Text.Text"=w4250) -> ()  [unwired: 2 in, 2 out]
                }
                frame 108 {
                  n3245 = property on="TITTLE" class="Str"("Caption.Text"=w4251) -> ()  [unwired: 2 in, 2 out]
                }
                frame 109 {
                  "String 30" <- w4252
                }
                frame 110 {
                  n3246 = property on="Test Date" class="Str"("Caption.Text"=w4253) -> ()  [unwired: 2 in, 2 out]
                  "String 31" <- w4253
                }
                frame 111 {
                  n3247 = property on="Sample ID" class="Str"("Caption.Text"=w4254) -> ()  [unwired: 2 in, 2 out]
                  "String 32" <- w4254
                }
                frame 112 {
                  n3248 = property on="Tested by" class="Str"("Caption.Text"=w4255) -> ()  [unwired: 2 in, 2 out]
                  "String 33" <- w4255
                }
                frame 113 {
                  n3249 = property on="System Configured Printers 2" class="Arr (strict)"("Caption.Text"=w4256) -> ()  [unwired: 2 in, 2 out]
                }
                frame 114 {
                  n3250 = property on="Selected Printer" class="Str"("Caption.Text"=w4257) -> ()  [unwired: 2 in, 2 out]
                }
                frame 115 {
                  n3251 = property on="Select Printer 3" class="DigNum (strict)"("Caption.Text"=w4258) -> ()  [unwired: 2 in, 2 out]
                }
                frame 116 {
                  n3252 = property on="Print" class="Bool (strict)"("Boolean Text.Text"=w4259) -> ()  [unwired: 2 in, 2 out]
                }
                frame 117 {
                  "String 41" <- w4260
                }
                frame 118 {
                  n3253 = property on="tested by" class="Str"("Caption.Text"=w4261) -> ()  [unwired: 2 in, 2 out]
                }
                frame 119 {
                }
                frame 120 {
                  n3254 = property on="Export" class="Bool (strict)"("Boolean Text.Text"=w4262) -> ()  [unwired: 2 in, 2 out]
                }
                frame 121 {
                }
                frame 122 {
                }
                frame 123 {
                  n3255 = property on="Select File Type" class="Enum (strict)"("Caption.Text"=w4265) -> ()  [unwired: 2 in, 2 out]
                }
                frame 124 {
                  n3256 = property on="s.NO" class="Str"("Caption.Text"=w4266) -> ()  [unwired: 2 in, 2 out]
                  "String 45" <- w4266
                }
                frame 125 {
                  n3257 = property on="trip1 8" class="Bool (strict)"("Boolean Text.Text"=w4267) -> ()  [unwired: 2 in, 2 out]
                }
                frame 126, Default {
                }
              }
            }
          }
          frame #1 {
            w4275 = TRUE ("Visible")
            n3258 = local read "S 91"() -> (w4292:string)
            n3259 = local read "S 90"() -> (w4291:string)
            n3260 = local read "S 88"() -> (w4290:string)
            n3261 = property on="File Path" class="Path"("Caption.Text"=w4291) -> ()  [unwired: 2 in, 2 out]
            n3262 = local read "S 71"() -> (w4285:string)
            n3263 = local read "S 86"() -> (w4287:string)
            n3264 = local read "S 85"() -> (w4288:string)
            n3265 = local read "S 87"() -> (w4286:string)
            n3266 = local read "S 84"() -> (w4289:string)
            n3267 = local read "S 103"() -> (w4274:string)
            n3268 = local read "S 104"() -> (w4273:string)
            n3269 = property on="Password" class="Str"("Caption.Text"=w4288) -> ()  [unwired: 2 in, 2 out]
            n3270 = property on="EDIT" class="Bool (strict)"("Boolean Text.Text"=w4285) -> ()  [unwired: 2 in, 2 out]
            n3271 = property on="SAVE" class="Bool (strict)"("Boolean Text.Text"=w4289) -> ()  [unwired: 2 in, 2 out]
            n3272 = Build Array(w4274, w4273) -> (w4272:string[])
            n3273 = property on="Heater Button" class="Bool (strict)"("Strings [4]"=w4272) -> ()  [unwired: 2 in, 2 out]
            n3274 = local read "S 92"() -> (w4284:string)
            n3275 = local read "S 93"() -> (w4283:string)
            n3276 = local read "S 105"() -> (w4270:string)
            n3277 = local read "S 106"() -> (w4269:string)
            n3278 = Build Array(w4284, w4283) -> ()  [unwired: 1 out]
            n3279 = Build Array(w4270, w4269) -> (w4271:string[])
            n3280 = local read "S 95"() -> (w4281:string)
            n3281 = local read "S 94"() -> (w4282:string)
            n3282 = local read "bs"() -> (w4297:string)
            n3283 = local read "as"() -> (w4298:string)
            n3284 = property on="Humidity" class="Bool (strict)"("Strings [4]"=w4271) -> ()  [unwired: 2 in, 2 out]
            n3285 = Concatenate Strings(w4297, "\r", w4298) -> ()  [unwired: 1 out]
            n3286 = property on="Rh After" class="DigNum (strict)"("Caption.Size to Text?"=TRUE ("Caption.Size to Text")) -> ()  [unwired: 2 in, 2 out]
            n3287 = local read "S 48"() -> (w4321:string)
            n3288 = local read "S 50"() -> (w4319:string)
            n3289 = local read "S 51"() -> (w4318:string)
            n3290 = local read "S 49"() -> (w4320:string)
            n3291 = local read "S 52"() -> (w4317:string)
            n3292 = local read "as"() -> (w4302:string)
            n3293 = local read "bs"() -> (w4303:string)
            n3294 = local read "S 56"() -> (w4316:string)
            n3295 = local read "S 57"() -> (w4315:string)
            n3296 = local read "S 58"() -> (w4314:string)
            n3297 = local read "S 59"() -> (w4313:string)
            n3298 = property on="OPEN" class="Bool (strict)"("Boolean Text.Text"=w4317) -> ()  [unwired: 2 in, 2 out]
            n3299 = property on="OPEN 1" class="Bool (strict)"("Boolean Text.Text"=w4321) -> ()  [unwired: 2 in, 2 out]
            n3300 = property on="OPEN 2" class="Bool (strict)"("Boolean Text.Text"=w4320) -> ()  [unwired: 2 in, 2 out]
            n3301 = property on="OPEN 3" class="Bool (strict)"("Boolean Text.Text"=w4319) -> ()  [unwired: 2 in, 2 out]
            n3302 = property on="OPEN 4" class="Bool (strict)"("Boolean Text.Text"=w4318) -> ()  [unwired: 2 in, 2 out]
            n3303 = Concatenate Strings(w4303, "\r", w4302) -> ()  [unwired: 1 out]
            n3304 = local read "S 102"() -> (w4276:string)
            n3305 = property on="КОФ1" class="DigNum (strict)"("Caption.Text"=w4316) -> ()  [unwired: 2 in, 2 out]
            n3306 = local read "S 98"() -> (w4280:string)
            n3307 = local read "S 99"() -> (w4279:string)
            n3308 = local read "S 100"() -> (w4278:string)
            n3309 = local read "S 101"() -> (w4277:string)
            n3310 = property on="КОФ2" class="DigNum (strict)"("Caption.Text"=w4315) -> ()  [unwired: 2 in, 2 out]
            n3311 = property on="КОФ3" class="DigNum (strict)"("Caption.Text"=w4314) -> ()  [unwired: 2 in, 2 out]
            n3312 = property on="КОФ4" class="DigNum (strict)"("Caption.Text"=w4313) -> ()  [unwired: 2 in, 2 out]
            n3313 = local read "bs"() -> (w4301:string)
            n3314 = local read "as"() -> (w4300:string)
            n3315 = local read "S 60"() -> (w4312:string)
            n3316 = local read "S 54"() -> (w4322:string)
            n3317 = Concatenate Strings(w4301, "\r", w4300) -> ()  [unwired: 1 out]
            n3318 = Concatenate Strings(w4322, w4312) -> ()  [unwired: 1 out]
            n3319 = local read "S 77"() -> (→"String 43":string)
            n3320 = local read "S 76"() -> (w4295:string)
            n3321 = local read "S 78"() -> (w4294:string)
            n3322 = local read "S 71"() -> (w4306:string)
            n3323 = local read "S 66"() -> (w4311:string)
            n3324 = local read "S 67"() -> (w4310:string)
            n3325 = local read "S 68"() -> (w4309:string)
            n3326 = local read "S 69"() -> (w4308:string)
            n3327 = local read "S 70"() -> (w4307:string)
            n3328 = property on="AIR TEMP" class="DigNum (strict)"("Caption.Text"=w4294) -> ()  [unwired: 2 in, 2 out]
            n3329 = property on="Set Strk" class="DigNum (strict)"("Caption.Text"=w4295) -> ()  [unwired: 2 in, 2 out]
            n3330 = property on="SPEED OUT:" class="DigNum (strict)"("Caption.Text"=w4309) -> ()  [unwired: 2 in, 2 out]
            n3331 = property on="EDIT" class="Bool (strict)"("Boolean Text.Text"=w4306) -> ()  [unwired: 2 in, 2 out]
            n3332 = local read "S 79"() -> (w4293:string)
          }
          frame #2 {
          }
        }
        n3333 = local write "Lan flag"(10.0 ("Lan flag")) -> ()
      }
      frame Enabled {
      }
    }
    n3334 = Wait (ms)(milliseconds to wait=u32 2000) -> ()  [unwired: 1 out]
    n3335 = local read "Quit"() -> (w4096:bool)
  }
  n3336 = while {
    shift-right: [w4328] -> _
    shift-left: _ -> [w4329]
    shift-right: [w4326] -> _
    shift-left: T18 {"Read Heave and Surge"="", "Bytes at Heave Port"=0.0, "Heave and Surge COM Port:"="COM9", "Com Port 2"="COM7", "Residual Due"="", "Heave COM Status 2"=TRUE, "Heave COM Status"=TRUE, "Port 2"=TRUE, "Sway PPR"=6400.0, "Surge PPR"=6400.0, "Heave PPR"=6400.0, "Sway Pitch"=2.0, "Surge Pitch"=3.0, "Heave Pitch"=4.0, "Sway Pulses/mm"=320.0, "Surge Pulses/mm"=1600.0, "Heave Pulses/mm"=1600.0, "inner loop"=0.0, "Read Heave and Surge 2"="", "String 36"="", "Write S"=FALSE, "WriteCC1"=[""], "Heave COM Loop"=0, "LastCom"="", "EXIT"=FALSE, "Error Heave"={"status"=TRUE, "code"=-1073807343, "source"=""}} -> [w4325]
    shift-right: [w4323] -> _
    shift-left: enum16{"init", "MAIN", "Panel Close"}."init" -> [w4324]
    stop <- w4327 stop-if-true
    # "HUMIDITY LOOP LOGIC"
    n3337 = case shown="\"MAIN\"" w4324 {
      tunnel: w4329 -> [w4343 w4362 w4417 w4419]
      tunnel: [w4338 w4366 w4417 w4419] -> w4328
      tunnel: [_ _ TRUE _] -> w4327
      tunnel: [w4335 w4364 w4415 w4418] -> w4326
      tunnel: w4325 -> [w4340 w4361 w4415 w4418]
      tunnel: [enum16{"init", "MAIN", "Panel Close"}."MAIN" w4356 _ _] -> w4323
      frame "init" {
        n3338 = local read "C3 :"() -> (w4330:refnum<visa-resource-name>)
        n3339 = Bundle By Name(cluster=w4340, "Heave and Surge COM Port:"=w4330) -> (w4339:T18)
        n3340 = call "Instrument fgv uno.vi"("Enum"=T31."INIT", "error in (no error) 2"=w4343, "INPUT"=w4339) -> ("error"=w4341:errorcluster, "output"=w4337:T18)  [unwired: 6 in, 1 out]
        n3341 = case shown="Error" w4341 {
          selector: w4341 -> [w4345 _]
          tunnel: [w4345 w4349] -> w4338
          tunnel: w4337 -> [w4344 w4347]
          tunnel: [w4344 w4346] -> w4336
          frame No Error {
          }
          frame Error {
            n3342 = call "Instrument fgv uno.vi"("Enum"=T31."ERROR INIT", "INPUT"=w4347) -> ("error"=w4350:errorcluster, "output"=w4346:T18)  [unwired: 7 in, 1 out]
            n3343 = call <vilib>:"Clear Errors.vi"("error in (no error)"=w4350) -> ("error out"=w4349:errorcluster)  [unwired: 5 in, 1 out]
          }
        }
        n3344 = local read "LastCom Humidity"() -> (w4333:string)
        n3345 = Unbundle By Name(w4336) -> ("Heave COM Status 2"=→"COM Status":bool, "Error Heave"=→"Error":errorcluster)  [unwired: 1 out]
        n3346 = Bundle By Name(cluster=w4336, "LastCom"=w4333) -> (w4335:T18)
      }
      frame "MAIN" {
        n3347 = Unbundle By Name(w4361) -> ("Com Port 2"=w4351:refnum<visa-resource-name>)
        n3348 = local read "C3 :"() -> (w4352:refnum<visa-resource-name>)
        n3349 = local write "COM Port Humidity :"(w4351) -> ()
        n3350 = Bundle By Name(cluster=w4361, "Heave and Surge COM Port:"=w4352) -> (w4360:T18)
        n3351 = Equal?(x=w4351, y=w4352) -> (x = y?=w4367:bool)
        n3352 = case shown="True" w4367 {
          tunnel: [w4371 w4388] -> w4366
          tunnel: w4362 -> [w4372 w4394]
          tunnel: w4360 -> [w4370 w4392]
          tunnel: [w4369 w4387] -> w4364
          frame False {
            n3353 = call <vilib>:"Clear Errors.vi"("error in (no error)"=w4372) -> ("error out"=w4368:errorcluster)  [unwired: 5 in, 1 out]
            n3354 = call "Instrument fgv uno.vi"("Enum"=T31."ERROR INIT", "error in (no error) 2"=w4368, "INPUT"=w4370) -> ("error"=w4374:errorcluster, "output"=w4369:T18)  [unwired: 6 in, 1 out]
            n3355 = call <vilib>:"Clear Errors.vi"("error in (no error)"=w4374) -> ("error out"=w4371:errorcluster)  [unwired: 5 in, 1 out]
          }
          frame True {
            n3356 = call "Instrument fgv uno.vi"("Enum"=T31."READ", "error in (no error) 2"=w4394, "INPUT"=w4392) -> ("error"=w4393:errorcluster, "output"=w4386:T18)  [unwired: 6 in, 1 out]
            n3357 = Bundle By Name(cluster=w4386, "String 36"="WRITE HUMIDITY") -> (w4385:T18)
            n3358 = case shown="True" "Write Humidity" {
              selector: "Write Humidity" -> [_ w4414]
              tunnel: w4393 -> [w4407 w4413]
              tunnel: [w4407 w4412] -> w4383
              tunnel: w4385 -> [w4406 w4410]
              tunnel: [w4406 w4409] -> w4382
              frame False {
              }
              frame True {
                n3359 = Not(x=w4414) -> (.not. x?=w4408:bool)
                n3360 = local write "Write Humidity"(w4408) -> ()
                n3361 = call "Instrument fgv uno.vi"("Enum"=T31."MANUAL WRITE", "error in (no error) 2"=w4413, "INPUT"=w4410) -> ("error"=w4412:errorcluster, "output"=w4409:T18)  [unwired: 6 in, 1 out]
              }
            }
            n3362 = Array Size(array="WriteHumidity") -> (size(s)=w4380:i32)
            n3363 = Greater Than 0?(x=w4380) -> (x > 0?=w4379:bool)
            n3364 = call "Instrument fgv uno.vi"("Enum"=T31."WRITE", "error in (no error) 2"=w4383, "WriteCC1"="WriteHumidity", "INPUT"=w4382) -> ("error"=w4390:errorcluster, "WriteCC1 2"=w4381:string[], "output"=w4389:T18)  [unwired: 5 in]
            n3365 = case shown="True" w4379 {
              tunnel: w4381 -> [_ w4396]
              frame False {
              }
              frame True {
                n3366 = local write "WriteHumidity"(w4396) -> ()
              }
            }
            n3367 = case shown="No Error" w4390 {
              selector: w4390 -> [w4397 w4400]
              tunnel: w4389 -> [w4398 w4405]
              tunnel: [w4398 w4404] -> w4387
              tunnel: [w4397 w4402] -> w4388
              frame No Error {
              }
              frame Error {
                n3368 = call <vilib>:"Clear Errors.vi"("error in (no error)"=w4400) -> ("error out"=w4399:errorcluster)  [unwired: 5 in, 1 out]
